vi "InputValues.vi"() -> ()   [LabVIEW 2016]
panel:
  out "Start":bool
  out "Select":bool
  out "RB":bool
  out "LB":bool
  out "Y":bool
  out "X":bool
  out "B":bool
  out "A":bool
  in  "Joystick Y":dbl(knob) scale=-1.0..1.0
  in  "Joystick X":dbl(knob) scale=-1.0..1.0
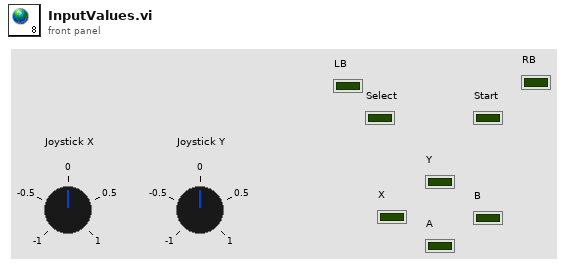
[diagram p1: front panel]
diagram:
